vi "PDC_GetMemImageData.vi"(0 "DeviceNo":u32, 1 "ColorType":enum16{"MONO", "COLOR"}(ring), 5 "ChildNo":u32, 7 "FrameNo":i32, 9 "BitDepth":u32, 11 "error in (no error)":errorcluster, 12 "Resolution":cluster{"Width":u32, "Height":u32}) -> (2 "Data(16Bit)":u16[](array[numeric]), 4 "ReturnValue":u32, 13 "Data(8Bit)":u8[](array[numeric]), 14 "ErrorCode":u32, 15 "error out":errorcluster)   [LabVIEW 2015]
doc: "This VI retrieves the recording image of the specified child device's current partition."
uses:
  PDCLIB.dll
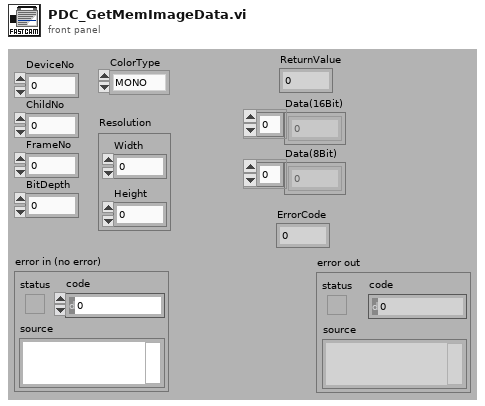
[diagram p1: front panel]
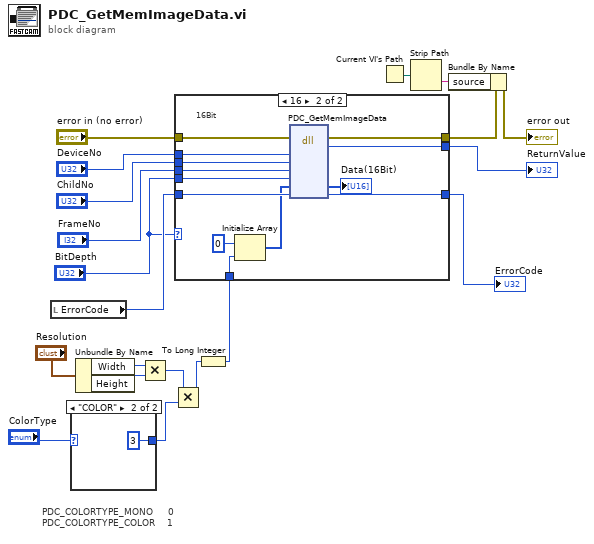
[diagram p0: block diagram]
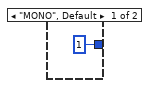
[diagram p2: hidden frame]
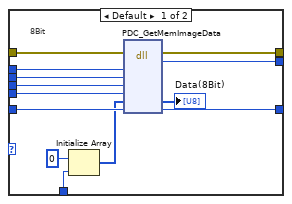
[diagram p3: hidden frame]
diagram:
  # "PDC_COLORTYPE_MONO\t\t\t\t\t0\nPDC_COLORTYPE_COLOR\t\t\t\t1"
  n1 = local read "ErrorCode"() -> (w18:u32)
  n2 = case shown="\"COLOR\"" "ColorType" {
    tunnel: [u32 1 ("y") u32 3 ("y")] -> w7
    frame "MONO", Default {
    }
    frame "COLOR" {
    }
  }
  n3 = Unbundle By Name("Resolution") -> ("Width"=w11:u32, "Height"=w10:u32)
  n4 = Multiply(x=w11, y=w10) -> (x*y=w13:u32)
  n5 = Multiply(x=w13, y=w7) -> (x*y=w12:u32)
  n6 = To Long Integer(number=w12) -> (32bit integer=w2:i32)
  n7 = case shown="16" "BitDepth" {
    tunnel: [w35 w48] -> w20
    tunnel: [w34 w47] -> w4
    tunnel: "error in (no error)" -> [w33 w46]
    tunnel: w18 -> [w32 w45]
    tunnel: "DeviceNo" -> [w31 w44]
    tunnel: "ChildNo" -> [w30 w43]
    tunnel: [w29 w42] -> w15
    tunnel: "BitDepth" -> [w28 w41]
    tunnel: "FrameNo" -> [w27 w40]
    tunnel: w2 -> [w24 w38]
    frame Default {
      # "8Bit"
      n8 = Initialize Array(u8 0 ("—v‘f"), w24) -> (w23:u8[])
      n9 = dll-call lib="PDCLIB.dll" fn="PDC_GetMemImageData"(error in=w33, "nDeviceNo"=w31, "nChildNo"=w30, "nFrameNo"=w27, "nBitDepth"=w28, "pData"=w23, "pErrorCode"=w32) -> (error out=w34:errorcluster, "return type"=w35:u32, "pData"=→"Data(8Bit)":u8[], "pErrorCode"=w29:u32)  [unwired: 6 in, 1 out]
    }
    frame 16 {
      # "16Bit"
      n10 = Initialize Array(u16 0 ("—v‘f"), w38) -> (w37:u16[])
      n11 = dll-call lib="PDCLIB.dll" fn="PDC_GetMemImageData"(error in=w46, "nDeviceNo"=w44, "nChildNo"=w43, "nFrameNo"=w40, "nBitDepth"=w41, "pData"=w37, "pErrorCode"=w45) -> (error out=w47:errorcluster, "return type"=w48:u32, "pData"=→"Data(16Bit)":u16[], "pErrorCode"=w42:u32)  [unwired: 6 in, 1 out]
    }
  }
  "ReturnValue" <- w20
  "ErrorCode" <- w15
  n12 = Current VI's Path() -> (path=w5:path)
  n13 = Strip Path(path=w5) -> (name=w6:string)  [unwired: 1 out]
  n14 = Bundle By Name(cluster=w4, "source"=w6) -> (→"error out":errorcluster)
